vi "JYInitFW.vi"(8 "error in (no error)":errorcluster, 9 "Force?":bool, 11 "FW Unique ID":string="FW1") -> (0 "error out":errorcluster, 1 "Emulating":bool, 2 "Initialized":bool, 3 "FW RefNum Out":refnum<k7>)   [LabVIEW 2012]
doc: "Initializes the internal Filter Wheel using it's Unique ID (FW1,FW2,...)."
panel:
  out "Initialize?":bool=TRUE
  in  "FW RefNum In":refnum<k7>
  # "Yes"
  # "No"
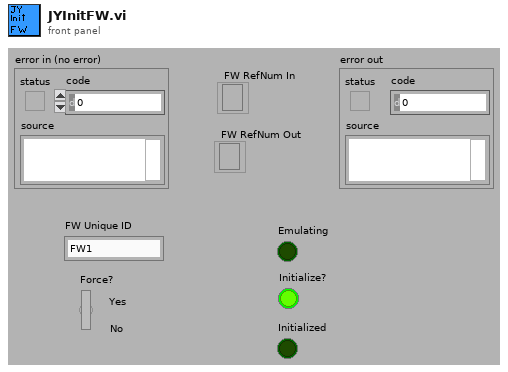
[diagram p1: front panel]
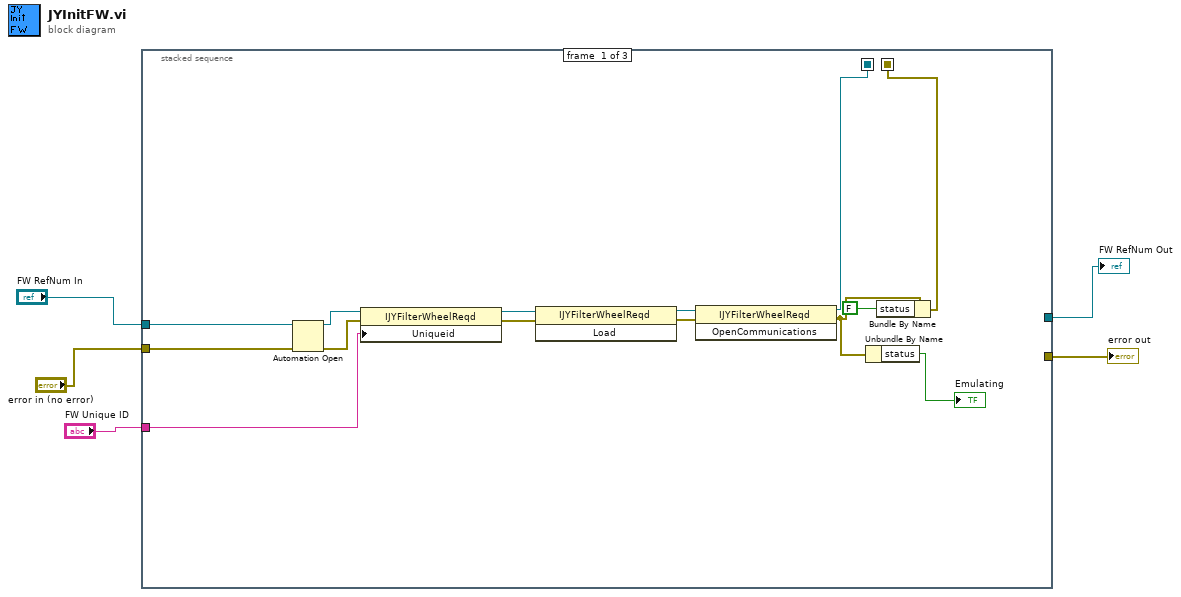
[diagram p0: block diagram]
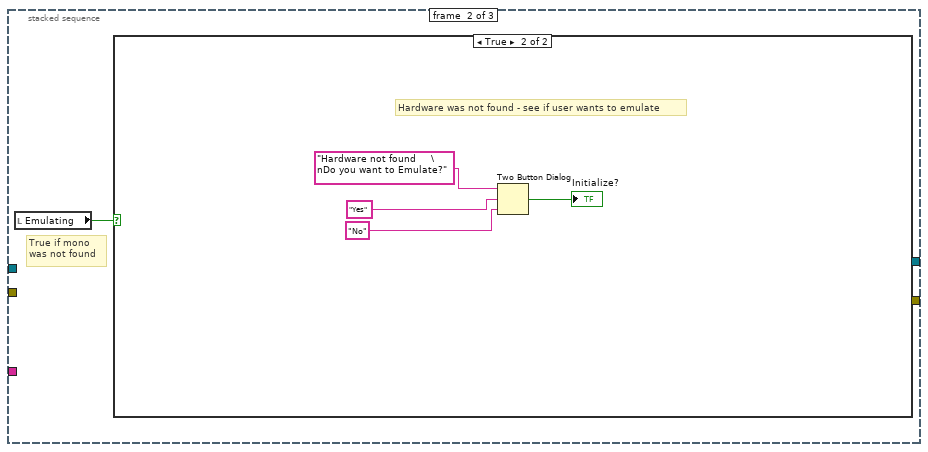
[diagram p2: hidden frame]
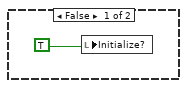
[diagram p3: hidden frame]
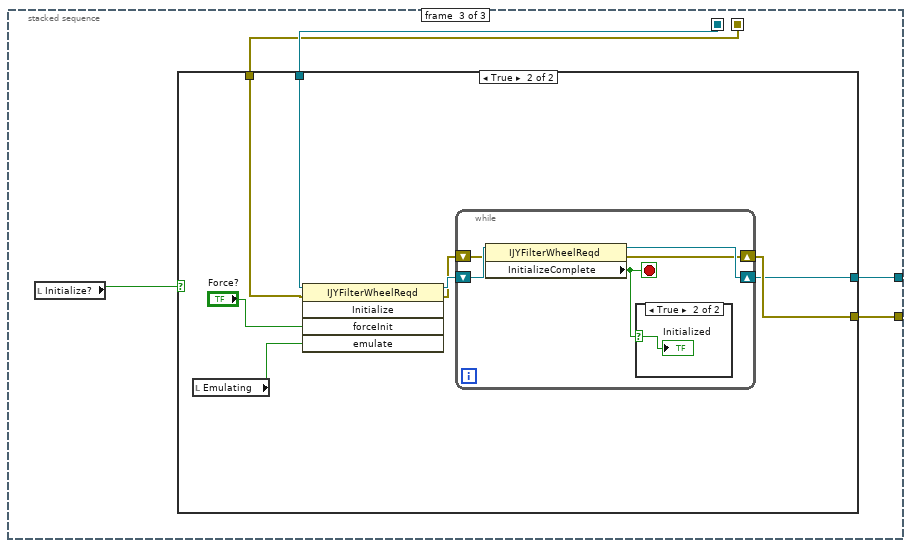
[diagram p4: hidden frame]
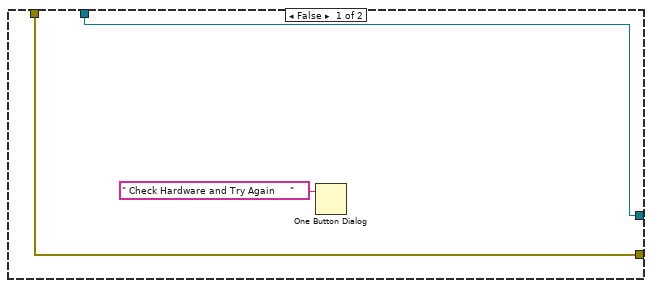
[diagram p5: hidden frame]
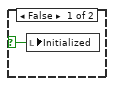
[diagram p6: hidden frame]
diagram:
  n1 = stacked-sequence {
    seq-local: [w7 _ _] -> [_ _ w29]
    seq-local: [w6 _ _] -> [_ _ w28]
    tunnel: "FW RefNum In" -> [w19 _ _]
    tunnel: "FW Unique ID" -> [w17 _ _]
    tunnel: "error in (no error)" -> [w8 _ _]
    tunnel: [_ _ w27] -> w2
    tunnel: [_ _ w26] -> w1
    frame #0 {
      n2 = Automation Open(error in (no error)=w8, Automation Refnum=w19) -> (Automation Refnum=w18:refnum<k7>, error out=w16:errorcluster)  [unwired: 2 out]
      n3 = property class="IJYFilterWheelReqd"(reference=w18, error in=w16, "Uniqueid"=w17) -> (reference out=w14:refnum<k7>, error out=w15:errorcluster)
      n4 = invoke class="IJYFilterWheelReqd" method="Load"(reference=w14, error in=w15) -> (reference out=w13:refnum<k7>, error out=w12:errorcluster)  [unwired: 1 in, 1 out]
      n5 = invoke class="IJYFilterWheelReqd" method="OpenCommunications"(reference=w13, error in=w12) -> (reference out=w7:refnum<k7>, error out=w11:errorcluster)  [unwired: 1 in, 1 out]
      n6 = Unbundle By Name(w11) -> ("status"=→"Emulating":bool)
      n7 = Bundle By Name(cluster=w11, "status"=FALSE) -> (w6:errorcluster)
    }
    frame #1 {
      # "True if mono\nwas not found"
      n8 = local read "Emulating"() -> (w20:bool)
      n9 = case shown="True" w20 {
        frame False {
          n10 = local write "Initialize?"(TRUE ("Initialize")) -> ()
        }
        frame True {
          # "Hardware was not found - see if user wants to emulate"
          n11 = Two Button Dialog(message="Hardware not found     \nDo you want to Emulate?", 1:"No" ("F button name (\"Cancel\")"), 2:"Yes" ("T button name (\"OK\")")) -> (T button?=→"Initialize?":bool)
        }
      }
    }
    frame #2 {
      n12 = local read "Initialize?"() -> (w30:bool)
      n13 = case shown="True" w30 {
        tunnel: w29 -> [w32 w39]
        tunnel: w28 -> [w31 w38]
        tunnel: [w31 w35] -> w27
        tunnel: [w32 w34] -> w26
        frame False {
          n14 = One Button Dialog(message=" Check Hardware and Try Again     ") -> ()  [unwired: 2 out]
        }
        frame True {
          n15 = local read "Emulating"() -> (w41:bool)
          n16 = invoke class="IJYFilterWheelReqd" method="Initialize"(reference=w39, error in=w38, "forceInit"="Force?", "emulate"=w41) -> (reference out=w37:refnum<k7>, error out=w36:errorcluster)  [unwired: 1 in, 3 out]
          n17 = while {
            shift-right: [w42] -> w35
            shift-left: w36 -> [w45]
            shift-right: [w43] -> w34
            shift-left: w37 -> [w46]
            stop <- w44 stop-if-true
            n18 = property class="IJYFilterWheelReqd"(reference=w46, error in=w45) -> (reference out=w43:refnum<k7>, error out=w42:errorcluster, "InitializeComplete"=w44:bool)
            n19 = case shown="True" w44 {
              selector: w44 -> [w47 w48]
              frame False {
                n20 = local write "Initialized"(w47) -> ()
              }
              frame True {
                "Initialized" <- w48
              }
            }
          }
        }
      }
    }
  }
  "error out" <- w2
  "FW RefNum Out" <- w1
